vi "Launch Root Analog Reader Actor.vi"(8 "error in (no error)":errorcluster, 10 "Analog Reader Actor":refnum<class "Analog Reader.lvclass">) -> (0 "error out":errorcluster, 1 "Analog Input Current Values":refnum<queue>, 2 "Actor's Enqueuer":refnum<class "Message Enqueuer.lvclass">)   [LabVIEW 2024, in "DAQmx Actor.lvlib" / "Analog Reader.lvclass"]
uses:
  Analog Reader.lvclass
  <vilib>/ActorFramework/Message Enqueuer/Message Enqueuer.lvclass
  Analog Reader Messages/Get High Speed Data Queue Msg/Get High Speed Data Queue Msg.lvclass/Get High Speed Data Queue Msg.ctl
  <vilib>/ActorFramework/Message Enqueuer/Message Enqueuer.lvclass/Message Enqueuer.ctl
  <vilib>/ActorFramework/Message Enqueuer/Enqueue.vi
  Analog Reader Messages/Get High Speed Data Queue Msg/Get High Speed Data Queue Msg.lvclass
  <vilib>/ActorFramework/Message Priority Queue/Priority Enqueue.vi
  Analog Reader.lvclass/Analog Reader.ctl
  <vilib>/ActorFramework/Actor/Actor.lvclass
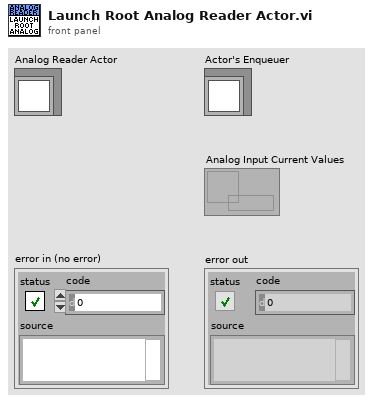
[diagram p1: front panel]
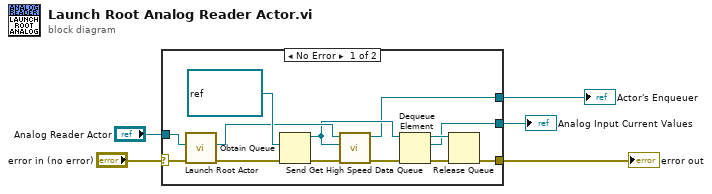
[diagram p0: block diagram]
diagram:
  n1 = case shown="No Error" "error in (no error)" {
    selector: "error in (no error)" -> [w6 w19]
    tunnel: "Analog Reader Actor" -> [w7 _]
    tunnel: [w10 w19] -> w4
    tunnel: [w9 _] -> w3
    tunnel: [w8 _] -> w2
    frame No Error {
      n2 = call <vilib>:"Launch Root Actor.vi"("error in (no error)"=w6, "Actor"=w7) -> ("error out"=w16:errorcluster, "Actor's Enqueuer"=w17:refnum<class "Message Enqueuer.lvclass">)  [unwired: 8 in]
      n3 = Obtain Queue(element data type=refnum<queue> refnum ("High Speed Data"), error in (no error)=w16) -> (queue out=w14:refnum<queue>, error out=w15:errorcluster)  [unwired: 3 in, 1 out]
      n4 = call "Send Get High Speed Data Queue.vi"("error in (no error)"=w15, "Queue of Queue"=w14, "Message Enqueuer"=w17) -> ("error out"=w13:errorcluster, "Message Enqueuer out"=w8:refnum<class "Message Enqueuer.lvclass">)  [unwired: 7 in]
      n5 = Dequeue Element(queue=w14, error in (no error)=w13) -> (queue out=w12:refnum<queue>, element=w9:refnum<queue>, error out=w11:errorcluster)  [unwired: 1 in, 1 out]
      n6 = Release Queue(queue=w12, error in (no error)=w11) -> (error out=w10:errorcluster)  [unwired: 1 in, 2 out]
    }
    frame Error {
    }
  }
  "error out" <- w4
  "Analog Input Current Values" <- w3
  "Actor's Enqueuer" <- w2
